vi "DSF.Engine.Transceiver.Tx.vi"(8 "error in (no error)":errorcluster, 10 "Transfer Group in":refnum<class "DSF.Engine.Transfer Group.lvclass">, 11 "GE Reflective Memory Transceiver in":refnum<class "DSF.Transceiver.GE Reflective Memory.lvclass">) -> (0 "error out":errorcluster, 2 "Transfer Group out":refnum<class "DSF.Engine.Transfer Group.lvclass">, 3 "GE Reflective Memory Transceiver out":refnum<class "DSF.Transceiver.GE Reflective Memory.lvclass">)   [LabVIEW 2017, in "DSF.Transceiver.GE Reflective Memory.lvlib" / "DSF.Transceiver.GE Reflective Memory.lvclass"]
uses:
  DSF.Transceiver.GE Reflective Memory.lvclass
  <vilib>/NI/GE Reflective Memory Driver/GE 5565PIORC.lvclass
  DSF Core/Built/Engine/DSF.Engine.lvlibp/Engine/Classes/Transfer/DSF.Engine.Transfer Group.lvclass
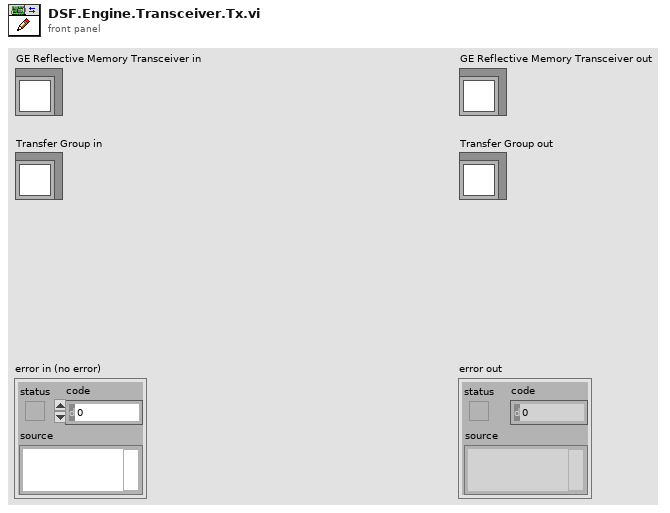
[diagram p1: front panel]
types:
  T1 = typedef "DSF.Transceiver.GE Reflective Memory.lvlib/DSF.Transceiver.GE Reflective Memory.lvclass/DSF.Transceiver.GE Reflective Memory.Transfer Group Parameters.ctl" = cluster{"DMA Transfer Specs":T2[]}
  T2 = typedef "GE 5565PIORC.lvclass/GE 5565PIORC.Typedef.DMA Transfer Spec.ctl" = cluster{"RFM offset":u32, "Block Descriptors":T3[]}
  T3 = typedef "GE 5565PIORC.lvclass/GE 5565PIORC.Typedef.DMA Block Descriptor.ctl" = cluster{"descriptor ptr (VISA)":u32, "descriptor ptr (RFM)":u32, "descriptor size":u32, "descriptor params":T4}
  T4 = typedef "GE 5565PIORC.lvclass/GE 5565PIORC.Typedef.DMA Block Descriptor Params.ctl" = cluster{"data ptr (lower)":u32, "data ptr (upper)":u32, "data size":u32, "next descriptor ptr":u32}
  T5 = typedef "GE 5565PIORC.lvclass/GE 5565PIORC.Typedef.DMA Wait Mode.ctl" = enum16{"Polling", "Interrupt"}
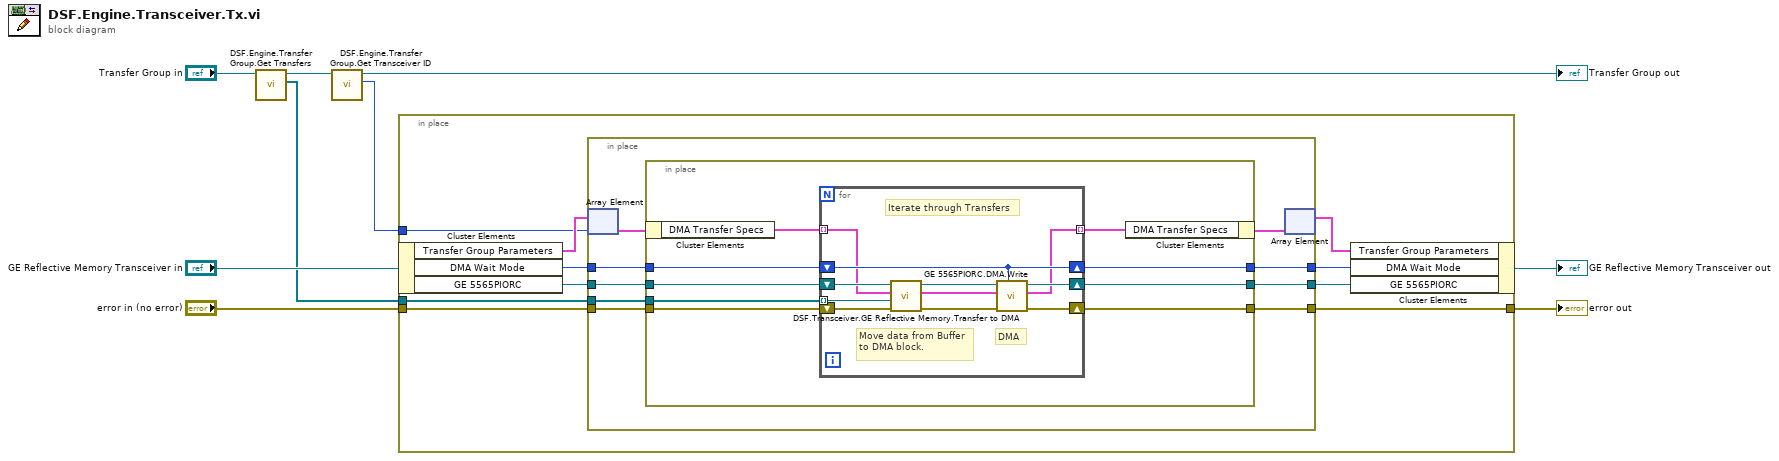
[diagram p0: block diagram]
diagram:
  n1 = call "DSF.Engine.Transfer Group.Get Transfers.vi"("Transfer Group in"="Transfer Group in") -> ("Transfers"=w4:refnum<class "DSF.Engine.Transfer.lvclass">[], "Transfer Group out"=w2:refnum<class "DSF.Engine.Transfer Group.lvclass">)  [unwired: 9 in]
  n2 = call "DSF.Engine.Transfer Group.Get Transceiver ID.vi"("Transfer Group in"=w2) -> ("transceiver id"=w5:i32, "Transfer Group out"=→"Transfer Group out":refnum<class "DSF.Engine.Transfer Group.lvclass">)  [unwired: 9 in]
  n3 = in-place {
    in-place-border: "error in (no error)" -> [w18]
    in-place-border: [w17] -> w8
    in-place-border: w5 -> [w12]
    in-place-border: w4 -> [w10]
    n4 = in-place-cluster #1("GE Reflective Memory Transceiver in") -> ("Transfer Group Parameters"=w13:T1[], "DMA Wait Mode"=w15:T5, "GE 5565PIORC"=w19:refnum<class "GE 5565PIORC.lvclass">)
    n5 = in-place {
      in-place-border: w19 -> [w28]
      in-place-border: w18 -> [w27]
      in-place-border: [w26] -> w17
      in-place-border: [w25] -> w16
      in-place-border: w15 -> [w24]
      in-place-border: [w23] -> w14
      in-place-border: w10 -> [w20]
      n6 = in-place-array #2(w13, w12) -> (w22:T1)
      n7 = in-place {
        in-place-border: w28 -> [w37]
        in-place-border: w27 -> [w36]
        in-place-border: [w31] -> w26
        in-place-border: [w35] -> w25
        in-place-border: w24 -> [w34]
        in-place-border: [w33] -> w23
        in-place-border: w20 -> [w29]
        n8 = in-place-cluster #3(w22) -> ("DMA Transfer Specs"=w32:T2[])
        n9 = for {
          shift-right: [w47] -> w35
          shift-left: w37 -> [w44]
          shift-right: [w48] -> w31
          shift-left: w36 -> [w43]
          shift-right: [w46] -> w33
          shift-left: w34 -> [w46]
          tunnel: w32 -> [w42] mode=indexing
          tunnel: [w45] -> w30 mode=indexing
          tunnel: w29 -> [w38] mode=indexing
          # "Iterate through Transfers"
          # "DMA"
          # "Move data from Buffer to DMA block."
          n10 = call "DSF.Transceiver.GE Reflective Memory.Transfer to DMA.vi"("error in (no error)"=w43, "Transfer in"=w38, "DMA Transfer Spec in"=w42, "GE 5565PIORC in"=w44) -> ("error out"=w39:errorcluster, "DMA Transfer Spec out"=w41:T2, "GE 5565PIORC out"=w40:refnum<class "GE 5565PIORC.lvclass">)  [unwired: 4 in, 1 out]
          n11 = call <vilib>:"GE 5565PIORC.DMA.Write.vi"("wait mode (polling)"=w46, "error in (no error)"=w39, "DMA Transfer Spec"=w41, "GE 5565PIORC in"=w40) -> ("error out"=w48:errorcluster, "DMA Transfer Spec dup"=w45:T2, "GE 5565PIORC out"=w47:refnum<class "GE 5565PIORC.lvclass">)  [unwired: 4 in, 1 out]
        }
        n12 = in-place-cluster #3("DMA Transfer Specs"=w30) -> (w21:T1)
      }
      n13 = in-place-array #2(w21) -> (w11:T1[])  [unwired: 1 out]
    }
    n14 = in-place-cluster #1("Transfer Group Parameters"=w11, "DMA Wait Mode"=w14, "GE 5565PIORC"=w16) -> (→"GE Reflective Memory Transceiver out":refnum<class "DSF.Transceiver.GE Reflective Memory.lvclass">)
  }
  "error out" <- w8
